vi "LSMcontroller_v60_PIzstage.vi"() -> ()   [LabVIEW 2015] (continued)
                n2600 = Unbundle By Name(w5604) -> ("Vto2P"=w5603:i32, "AOlines"=w5602:tag[])
                n2601 = local write "Vpockels"(w5598) -> ()
                n2602 = property on="Laserpower \n(%)" class="Slide (strict)"("Value"=w5600) -> ()  [unwired: 2 in, 2 out]
                n2603 = Index Array(array=w5602, index=w5603) -> (element=w5601:tag)
                n2604 = call-poly <vilib>:"DAQmx Create Virtual Channel.vi"("physical channels"=w5601) -> ("task out"=w5607:refnum<k21>, "error out"=w5606:errorcluster)  [unwired: 13 in]
                n2605 = call-poly <vilib>:"DAQmx Write.vi"("task/channels in"=w5607, "data"=w5598, "error in"=w5606) -> ("task out"=w5608:refnum<k21>, "error out"=w5609:errorcluster)  [unwired: 10 in, 1 out]
                n2606 = call <vilib>:"DAQmx Start Task.vi"("task/channels in"=w5608, "error in"=w5609) -> ("task out"=w5610:refnum<k21>, "error out"=w5611:errorcluster)  [unwired: 12 in]
                n2607 = call <vilib>:"DAQmx Stop Task.vi"("task/channels in"=w5610, "error in"=w5611) -> ("task out"=w5612:refnum<k21>, "error out"=w5613:errorcluster)  [unwired: 12 in]
                n2608 = call <vilib>:"DAQmx Clear Task.vi"("task in"=w5612, "error in"=w5613) -> ()  [unwired: 13 in, 1 out]
              }
            }
          }
          event "sealtest": Value Change {
            n2609 = event-data() -> ()  [unwired: 1 in, 6 out]
            n2610 = case shown="True" "sealtest" {
              frame False {
              }
              frame True {
                n2611 = stacked-sequence {
                  seq-local: [w5615 _ _ _ _ _] -> [_ w5648 _ w5700 _ _]
                  frame #0 {
                    n2612 = stacked-sequence {
                      tunnel: [_ w5627 _] -> w5615
                      frame #0 {
                        n2613 = call "2pparameters.vi"("command"="get") -> ("params out"=w5620:T11)  [unwired: 1 in]
                        n2614 = Unbundle By Name(w5620) -> ("autoshutter"=w5621:bool)
                        n2615 = local read "OCchecked?"() -> (w5618:bool)
                        n2616 = call "sealtestwfparams.vi"("command"="set") -> ()  [unwired: 6 in, 1 out]
                        n2617 = case shown="False" w5618 {
                          frame False {
                            n2618 = One Button Dialog(message="Is the OC gain correct?", button name ("OK")="ok") -> (true=w5622:bool)
                            n2619 = local write "OCchecked?"(w5622) -> ()
                          }
                          frame True {
                          }
                        }
                        n2620 = case shown="True" w5621 {
                          frame False {
                          }
                          frame True {
                            n2621 = call "shuttercontrol.vi"("command"="close") -> ()  [unwired: 1 in, 1 out]
                          }
                        }
                        n2622 = call "allAI-temp.vi"("command"=enum16{"get", "set", "clear", "append"}."clear") -> ()  [unwired: 3 in, 2 out]
                      }
                      frame #1 {
                        n2623 = call "sealtestwfparams.vi"("command"="get") -> ("Params out"=w5633:T24)  [unwired: 6 in]
                        n2624 = Unbundle By Name(w5633) -> ("AO parameters"=w5631:T25)
                        n2625 = Index Array(array=w5631, index=0) -> (element=w5630:T26)
                        n2626 = call "generateRampedSquareWave_fromAOparameters.vi"("AO params"=w5630) -> ("Waveform"=w5626:waveform(dbl), "wflength"=w5627:i32)
                        n2627 = Build Array(w5626) -> (w5629:waveform(dbl)[])
                        n2628 = call "waveformssealtestbuffer.vi"("AO wf in"=w5629, "command"="set") -> ()  [unwired: 1 out]
                      }
                      frame #2 {
                        n2629 = local read "Vholding (mV)"() -> (w5636:sgl)
                        n2630 = local read "Current Clamp"() -> (w5642:bool)
                        n2631 = local read "Voltage Clamp"() -> (w5641:bool)
                        n2632 = local read "OCgain"() -> (w5637:sgl)
                        n2633 = local read "CC_ICgain"() -> (w5640:dbl)
                        n2634 = local read "holdon"() -> (w5635:bool)
                        n2635 = call "patchparameters.vi"("command"="get") -> ("Params out"=w5644:T14)  [unwired: 1 in]
                        n2636 = Bundle By Name(cluster=w5644, "VC"=w5641, "CC"=w5642, "CC_icg (pA/mv)"=w5640, "VC_icg (mV/mV)"=10.0, "OCG (mV/pA)"=w5637, "OVG (mV/mV)"=0.1, "Vhold (mV)"=w5636, "holdon"=w5635) -> (w5643:T14)
                        n2637 = call "patchparameters.vi"("Params in"=w5643, "command"="set") -> ()  [unwired: 1 out]
                      }
                    }
                  }
                  frame #1 {
                    w5647 = 2
                    n2638 = call "patchparameters.vi"("command"="get") -> ("Params out"=w5655:T14)  [unwired: 1 in]
                    n2639 = Unbundle By Name(w5655) -> ("holdon"=w5654:bool, "Vhold (mV)"=w5653:sgl, "CC_icg (pA/mv)"=w5661:sgl, "CC"=w5659:bool, "VC_icg (mV/mV)"=w5660:sgl)
                    n2640 = Select(t=w5661, s=w5659, f=w5660) -> (s? t:f=w5662:sgl)
                    n2641 = To Single Precision Float(number=0.001 ("y")) -> (single precision float=w5663:sgl)
                    n2642 = Compound Arithmetic op=MULTIPLY(w5653, w5662, w5663) -> (w5657:sgl)
                    n2643 = case shown="False" w5654 {
                      tunnel: w5657 -> [_ w5675]
                      tunnel: [0.0 w5675] -> w5650
                      frame False {
                      }
                      frame True {
                      }
                    }
                    n2644 = Greater Than 0?(x=w5647) -> (x > 0?=w5649:bool)
                    n2645 = case shown="True" w5649 {
                      tunnel: w5648 -> [_ w5664]
                      tunnel: w5647 -> [_ w5667]
                      frame False {
                      }
                      frame True {
                        n2646 = Initialize Array(sgl 0.0 ("element"), w5667, w5664) -> (w5665:sgl[][])
                        n2647 = call "allAI-temp.vi"("array in"=w5665, "command"=enum16{"get", "set", "clear", "append"}."set") -> ()  [unwired: 2 in, 2 out]
                      }
                    }
                    n2648 = flat-sequence {
                      tunnel: w5648 -> [w5671]
                      tunnel: w5648 -> [w5670]
                      tunnel: [w5670] -> w5652
                      tunnel: [w5669] -> w5651
                      tunnel: w5650 -> [w5669]
                      tunnel: w5652 -> [w5673]
                      tunnel: w5651 -> [w5672]
                      frame #0 {
                        n2649 = call "prepAI_sealtest.vi"("samples per channel"=w5671) -> ()  [unwired: 2 in]
                      }
                      frame #1 {
                        n2650 = call "prepAO_sealtest.vi"("Vhold"=w5672, "samples per channel"=w5673) -> ()  [unwired: 1 in]
                      }
                    }
                  }
                  frame #2 {
                    n2651 = stacked-sequence {
                      frame #0 {
                        n2652 = call "tempconfigAO.vi"("command"="get") -> ("Temp Config out"=w5679:T27)  [unwired: 1 in]
                        n2653 = Unbundle By Name(w5679) -> ("AO"=w5680:refnum<k21>[], "E_AO"=w5681:errorcluster[])
                        n2654 = for {
                          tunnel: w5680 -> [w5689] mode=indexing
                          tunnel: w5681 -> [w5688] mode=indexing
                          tunnel: [w5687] -> w5683 mode=indexing
                          tunnel: [w5686] -> w5684 mode=indexing
                          n2655 = call <vilib>:"DAQmx Start Task.vi"("task/channels in"=w5689, "error in"=w5688) -> ("task out"=w5687:refnum<k21>, "error out"=w5686:errorcluster)  [unwired: 12 in]
                        }
                        n2656 = call "tempconfigAO.vi"("command"="get") -> ("Temp Config out"=w5682:T27)  [unwired: 1 in]
                        n2657 = Bundle By Name(cluster=w5682, "AO"=w5683, "E_AO"=w5684) -> (w5685:T27)
                        n2658 = call "tempconfigAO.vi"("Temp Config in"=w5685, "command"="set") -> ()  [unwired: 1 out]
                      }
                      frame #1 {
                        n2659 = call "tempconfigAI.vi"("command"="get") -> ("Temp Config out"=w5691:T28)  [unwired: 1 in]
                        n2660 = Unbundle By Name(w5691) -> ("AI"=w5696:refnum<k21>, "E_AI"=w5697:errorcluster)
                        n2661 = call <vilib>:"DAQmx Start Task.vi"("task/channels in"=w5696, "error in"=w5697) -> ("task out"=w5698:refnum<k21>, "error out"=w5699:errorcluster)  [unwired: 12 in]
                        n2662 = call "tempconfigAI.vi"("command"="get") -> ("Temp Config out"=w5693:T28)  [unwired: 1 in]
                        n2663 = Bundle By Name(cluster=w5693, "AI"=w5698, "E_AI"=w5699) -> (w5695:T28)
                        n2664 = call "tempconfigAI.vi"("Temp Config in"=w5695, "command"="set") -> ()  [unwired: 1 out]
                      }
                    }
                  }
                  frame #3 {
                    n2665 = while {
                      tunnel: w5700 -> [w5701]
                      stop <- w5702 stop-if-true
                      n2666 = local read "sealtest"() -> (w5705:bool)
                      n2667 = Not(x=w5705) -> (.not. x?=w5704:bool)
                      n2668 = case shown="False" w5704 {
                        tunnel: w5701 -> [w5706 _]
                        frame False {
                          n2669 = stacked-sequence {
                            seq-local: [_ _ _ w5745 _ _] -> [_ _ _ _ w5801 _]
                            seq-local: [w5707 _ _ _ _ _] -> [_ w5716 _ w5738 w5790 w5821]
                            tunnel: w5706 -> [_ _ w5724 _ w5789 _]
                            frame #0 {
                              n2670 = call "patchparameters.vi"("command"="get") -> ("Params out"=w5714:T14)  [unwired: 1 in]
                              n2671 = local read "Vholding (mV)"() -> (w5711:sgl)
                              n2672 = Unbundle By Name(w5714) -> ("Vhold (mV)"=w5710:sgl, "holdon"=w5713:bool)
                              n2673 = local read "holdon"() -> (w5712:bool)
                              n2674 = Not Equal?(x=w5711, y=w5710) -> (x != y?=w5709:bool)
                              n2675 = Not Equal?(x=w5713, y=w5712) -> (x != y?=w5708:bool)
                              n2676 = Or(x=w5709, y=w5708) -> (x .or. y?=w5707:bool)
                            }
                            frame #1 {
                              n2677 = case shown="True" w5716 {
                                frame False {
                                }
                                frame True {
                                n2678 = local read "Vholding (mV)"() -> (w5719:sgl)
                                n2679 = local read "holdon"() -> (w5717:bool)
                                n2680 = call "patchparameters.vi"("command"="get") -> ("Params out"=w5720:T14)  [unwired: 1 in]
                                n2681 = Bundle By Name(cluster=w5720, "Vhold (mV)"=w5719, "holdon"=w5717) -> (w5718:T14)
                                n2682 = call "patchparameters.vi"("Params in"=w5718, "command"="set") -> ()  [unwired: 1 out]
                                }
                              }
                            }
                            frame #2 {
                              n2683 = call "tempconfigAI.vi"("command"="get") -> ("Temp Config out"=w5734:T28)  [unwired: 1 in]
                              n2684 = Unbundle By Name(w5734) -> ("AI"=w5733:refnum<k21>, "E_AI"=w5732:errorcluster)
                              n2685 = call-poly <vilib>:"DAQmx Read.vi"("task/channels in"=w5733, "number of samples per channel"=w5724, "timeout"=10.0, "error in"=w5732) -> ("task out"=w5728:refnum<k21>, "data"=w5725:i16[][], "error out"=w5737:errorcluster)  [unwired: 9 in]
                              n2686 = call "tempconfigAI.vi"("command"="get") -> ("Temp Config out"=w5729:T28)  [unwired: 1 in]
                              n2687 = Bundle By Name(cluster=w5729, "AI"=w5728, "E_AI"=w5737) -> (w5736:T28)
                              n2688 = To Single Precision Float(number=w5725) -> (single precision float=w5727:sgl[][])
                              n2689 = call "tempconfigAI.vi"("Temp Config in"=w5736, "command"="set") -> ()  [unwired: 1 out]
                              n2690 = call "allAI-temp.vi"("array in"=w5727, "command"=enum16{"get", "set", "clear", "append"}."set") -> ()  [unwired: 2 in, 2 out]
                            }
                            frame #3 {
                              n2691 = case shown="True" w5738 {
                                frame False {
                                }
                                frame True {
                                n2692 = call "tempconfigAO.vi"("command"="get") -> ("Temp Config out"=w5778:T27)  [unwired: 1 in]
                                n2693 = Unbundle By Name(w5778) -> ("AO"=w5777:refnum<k21>[], "E_AO"=w5776:errorcluster[])
                                n2694 = call "tempconfigAI.vi"("command"="get") -> ("Temp Config out"=w5765:T28)  [unwired: 1 in]
                                n2695 = Unbundle By Name(w5765) -> ("AI"=w5766:refnum<k21>, "E_AI"=w5767:errorcluster)
                                n2696 = for {
                                tunnel: w5777 -> [w5782] mode=indexing
                                tunnel: w5776 -> [w5781] mode=indexing
                                tunnel: [w5780] -> w5772 mode=indexing
                                n2697 = call <vilib>:"DAQmx Stop Task.vi"("task/channels in"=w5782, "error in"=w5781) -> ("task out"=w5783:refnum<k21>, "error out"=w5784:errorcluster)  [unwired: 12 in]
                                n2698 = call <vilib>:"DAQmx Clear Task.vi"("task in"=w5783, "error in"=w5784) -> ("error out"=w5780:errorcluster)  [unwired: 13 in]
                                }
                                n2699 = call <vilib>:"DAQmx Stop Task.vi"("task/channels in"=w5766, "error in"=w5767) -> ("task out"=w5763:refnum<k21>, "error out"=w5762:errorcluster)  [unwired: 12 in]
                                n2700 = call <vilib>:"DAQmx Clear Task.vi"("task in"=w5763, "error in"=w5762) -> ("error out"=w5761:errorcluster)  [unwired: 13 in]
                                n2701 = call "tempconfigAO.vi"("command"="get") -> ("Temp Config out"=w5773:T27)  [unwired: 1 in]
                                n2702 = Bundle By Name(cluster=w5773, "E_AO"=w5772) -> (w5771:T27)
                                n2703 = call "tempconfigAI.vi"("command"="get") -> ("Temp Config out"=w5769:T28)  [unwired: 1 in]
                                n2704 = Bundle By Name(cluster=w5769, "E_AI"=w5761) -> (w5760:T28)
                                n2705 = call "tempconfigAO.vi"("Temp Config in"=w5771, "command"="set") -> ()  [unwired: 1 out]
                                n2706 = call "tempconfigAI.vi"("Temp Config in"=w5760, "command"="set") -> ()  [unwired: 1 out]
                                }
                              }
                              n2707 = call "allAI-temp.vi"("command"=enum16{"get", "set", "clear", "append"}."get") -> ("array out"=w5742:sgl[][])  [unwired: 3 in, 1 out]
                              n2708 = call "tempconfigAI.vi"("command"="get") -> ("Temp Config out"=w5755:T28)  [unwired: 1 in]
                              n2709 = call "tempconfigAI.vi"("command"="get") -> ("Temp Config out"=w5757:T28)  [unwired: 1 in]
                              n2710 = Unbundle By Name(w5755) -> ("header"=w5753:dbl[])
                              n2711 = Unbundle By Name(w5757) -> ("header"=w5759:dbl[])
                              n2712 = Index Array(array=w5742, index (row) #1=1 ("index (row)"), index (row) #2=0 ("index (row)")) -> (element #1=w5740:sgl[], element #2=w5739:sgl[])  [unwired: 2 in]
                              n2713 = local read "OCgain"() -> (w5747:sgl)
                              n2714 = call "Unscaledtoscaled.vi"("Unscaled Data"=w5740, "Header Information"=w5753) -> ("Array"=w5752:sgl[])  [unwired: 1 in]
                              n2715 = call "Unscaledtoscaled.vi"("Unscaled Data"=w5739, "Header Information"=w5759) -> ("Array"=w5756:sgl[])  [unwired: 1 in]
                              n2716 = Multiply(x=w5752, y=0.1) -> (x*y=w5749:dbl[])
                              n2717 = Divide(x=w5756, y=w5747) -> (x/y=w5748:sgl[])
                              n2718 = Build Array(w5749, w5748) -> (w5751:dbl[][])
                              n2719 = Multiply(x=w5751, y=1000.0) -> (x*y=w5745:dbl[][])
                              "Patch readout" <- w5745
                            }
                            frame #4 {
                              n2720 = case shown="True" w5790 {
                                tunnel: w5789 -> [_ w5802]
                                frame False {
                                }
                                frame True {
                                n2721 = call "patchparameters.vi"("command"="get") -> ("Params out"=w5806:T14)  [unwired: 1 in]
                                n2722 = Unbundle By Name(w5806) -> ("holdon"=w5805:bool, "Vhold (mV)"=w5804:sgl, "CC_icg (pA/mv)"=w5812:sgl, "CC"=w5810:bool, "VC_icg (mV/mV)"=w5811:sgl)
                                n2723 = Select(t=w5812, s=w5810, f=w5811) -> (s? t:f=w5813:sgl)
                                n2724 = To Single Precision Float(number=0.001 ("y")) -> (single precision float=w5814:sgl)
                                n2725 = Compound Arithmetic op=MULTIPLY(w5804, w5813, w5814) -> (w5808:sgl)
                                n2726 = case shown="True" w5805 {
                                tunnel: w5808 -> [_ w5819]
                                tunnel: [0.0 w5819] -> w5803
                                frame False {
                                }
                                frame True {
                                }
                                }
                                n2727 = flat-sequence {
                                tunnel: w5802 -> [w5815]
                                tunnel: w5803 -> [w5817]
                                tunnel: w5802 -> [w5816]
                                frame #0 {
                                n2728 = call "prepAI_sealtest.vi"("samples per channel"=w5815) -> ()  [unwired: 2 in]
                                }
                                frame #1 {
                                n2729 = call "prepAO_sealtest.vi"("Vhold"=w5817, "samples per channel"=w5816) -> ()  [unwired: 1 in]
                                }
                                }
                                }
                              }
                              n2730 = call "sealtestwfparams.vi"("command"="get") -> ("Params out"=w5795:T24)  [unwired: 6 in]
                              n2731 = Unbundle By Name(w5795) -> ("AO parameters"=w5796:T25)
                              n2732 = Index Array(array=w5796, index=0) -> (element=w5798:T26)
                              n2733 = Unbundle By Name(w5798) -> ("Cycles"=w5793:dbl, "Start amplitude (V)"=w5792:dbl, "Sampling frequency (Hz)"=w5791:dbl)
                              n2734 = local read "fitpoints"() -> (w5799:dbl)
                              n2735 = script code="V=data(1,:);\nI=data(2,:);\ntres=mean(V);\nspc=(nsamp./ncyc);\nV=V(spc+1:end-spc);\nI=I(spc+1:end-spc);\ndV=mean(V(V>tres))-mean(V(V<tres))\nIcyc=reshape(I,[spc ncyc-2]);\nIcyc=Icyc';\nIcyc=mean(Icyc,1);\ndIss=mean(Icyc(floor(spc*0.15):floor(spc/2)-2))-mean(Icyc(spc*0.65:spc-2))\nRm=dV*1e3/dIss;\n[maxi,ind]=max(Icyc);\nIfit=Icyc(ind+1:ind+1+points-1)-0.5*(mean(Icyc(floor(spc*0.15):floor(spc/2)-2))+mean(Icyc(spc*0.65:spc-2)))\nt=(3:points-1+3)./srate*1000;\nt=t';\nIfit=Ifit';\nc=fit(t,Ifit, 'exp1');\ncoeffs=coeffvalues(c);\nIa=coeffs(1);\nRa=dV*1e3./Ia/2;\ntau=-1./coeffs(2);\ncap=tau/Ra*1000;"("data"=w5801, "nsamp"=w5789, "ncyc"=w5793, "maxV"=w5792, "points"=w5799, "srate"=w5791) -> ("cap"=w5788:dbl, "Ra"=w5787:dbl, "Icyc"=w5786:dbl[], "Rm"=w5785:dbl)  [unwired: 1 in, 1 out]
                              n2736 = local read "set as Rp?"() -> (w5800:bool)
                              n2737 = local write "Cmembrane"(w5788) -> ()
                              n2738 = local write "Rmembrane (MOhm)"(w5785) -> ()
                              n2739 = local write "Racces (MOhm)"(w5787) -> ()
                              n2740 = case shown="True" w5800 {
                                tunnel: w5785 -> [_ w5820]
                                frame False {
                                }
                                frame True {
                                n2741 = local write "Rpipette (MOhm)"(w5820) -> ()
                                }
                              }
                              n2742 = local write "Ifit"(w5786) -> ()
                            }
                            frame #5 {
                              n2743 = local read "set as Rp?"() -> (w5822:bool)
                              n2744 = case shown="True" w5821 {
                                frame False {
                                }
                                frame True {
                                n2745 = stacked-sequence {
                                frame #0 {
                                n2746 = call "tempconfigAO.vi"("command"="get") -> ("Temp Config out"=w5829:T27)  [unwired: 1 in]
                                n2747 = Unbundle By Name(w5829) -> ("AO"=w5828:refnum<k21>[], "E_AO"=w5827:errorcluster[])
                                n2748 = for {
                                tunnel: w5828 -> [w5836] mode=indexing
                                tunnel: w5827 -> [w5835] mode=indexing
                                tunnel: [w5834] -> w5825 mode=indexing
                                tunnel: [w5833] -> w5824 mode=indexing
                                n2749 = call <vilib>:"DAQmx Start Task.vi"("task/channels in"=w5836, "error in"=w5835) -> ("task out"=w5834:refnum<k21>, "error out"=w5833:errorcluster)  [unwired: 12 in]
                                }
                                n2750 = call "tempconfigAO.vi"("command"="get") -> ("Temp Config out"=w5826:T27)  [unwired: 1 in]
                                n2751 = Bundle By Name(cluster=w5826, "AO"=w5825, "E_AO"=w5824) -> (w5823:T27)
                                n2752 = call "tempconfigAO.vi"("Temp Config in"=w5823, "command"="set") -> ()  [unwired: 1 out]
                                }
                                frame #1 {
                                n2753 = call "tempconfigAI.vi"("command"="get") -> ("Temp Config out"=w5838:T28)  [unwired: 1 in]
                                n2754 = Unbundle By Name(w5838) -> ("AI"=w5843:refnum<k21>, "E_AI"=w5844:errorcluster)
                                n2755 = call <vilib>:"DAQmx Start Task.vi"("task/channels in"=w5843, "error in"=w5844) -> ("task out"=w5845:refnum<k21>, "error out"=w5846:errorcluster)  [unwired: 12 in]
                                n2756 = call "tempconfigAI.vi"("command"="get") -> ("Temp Config out"=w5840:T28)  [unwired: 1 in]
                                n2757 = Bundle By Name(cluster=w5840, "AI"=w5845, "E_AI"=w5846) -> (w5842:T28)
                                n2758 = call "tempconfigAI.vi"("Temp Config in"=w5842, "command"="set") -> ()  [unwired: 1 out]
                                }
                                }
                                }
                              }
                              n2759 = case shown="True" w5822 {
                                frame False {
                                }
                                frame True {
                                n2760 = local write "set as Rp?"(FALSE ("set as Rp?")) -> ()
                                }
                              }
                            }
                          }
                        }
                        frame True {
                        }
                      }
                      n2761 = local read "sealtest"() -> (w5703:bool)
                      n2762 = Not(x=w5703) -> (.not. x?=w5702:bool)
                    }
                  }
                  frame #4 {
                    n2763 = call "tempconfigAO.vi"("command"="get") -> ("Temp Config out"=w5873:T27)  [unwired: 1 in]
                    n2764 = Unbundle By Name(w5873) -> ("AO"=w5872:refnum<k21>[], "E_AO"=w5871:errorcluster[])
                    n2765 = call "configuration.vi"("command"="get") -> ("config out"=w5854:T12)  [unwired: 2 in, 1 out]
                    n2766 = call "tempconfigAI.vi"("command"="get") -> ("Temp Config out"=w5860:T28)  [unwired: 1 in]
                    n2767 = Unbundle By Name(w5854) -> ("Device 1 sampleclock out"=w5851:tag, "Device 1 Starttrigger out"=w5850:tag)
                    n2768 = Unbundle By Name(w5860) -> ("AI"=w5861:refnum<k21>, "E_AI"=w5862:errorcluster)
                    n2769 = for {
                      tunnel: w5872 -> [w5877] mode=indexing
                      tunnel: w5871 -> [w5876] mode=indexing
                      tunnel: [w5875] -> w5867 mode=indexing
                      n2770 = call <vilib>:"DAQmx Stop Task.vi"("task/channels in"=w5877, "error in"=w5876) -> ("task out"=w5878:refnum<k21>, "error out"=w5879:errorcluster)  [unwired: 12 in]
                      n2771 = call <vilib>:"DAQmx Clear Task.vi"("task in"=w5878, "error in"=w5879) -> ("error out"=w5875:errorcluster)  [unwired: 13 in]
                    }
                    n2772 = call <vilib>:"DAQmx Stop Task.vi"("task/channels in"=w5861, "error in"=w5862) -> ("task out"=w5858:refnum<k21>, "error out"=w5857:errorcluster)  [unwired: 12 in]
                    n2773 = call <vilib>:"DAQmx Disconnect Terminals.vi"("source terminal"=tag "/Dev1/ai/SampleClock", "destination terminal"=w5851) -> ("error out"=w5848:errorcluster)  [unwired: 13 in]
                    n2774 = call <vilib>:"DAQmx Clear Task.vi"("task in"=w5858, "error in"=w5857) -> ("error out"=w5856:errorcluster)  [unwired: 13 in]
                    n2775 = call "tempconfigAO.vi"("command"="get") -> ("Temp Config out"=w5868:T27)  [unwired: 1 in]
                    n2776 = Bundle By Name(cluster=w5868, "E_AO"=w5867) -> (w5866:T27)
                    n2777 = call "tempconfigAI.vi"("command"="get") -> ("Temp Config out"=w5864:T28)  [unwired: 1 in]
                    n2778 = Bundle By Name(cluster=w5864, "E_AI"=w5856) -> (w5855:T28)
                    n2779 = call "tempconfigAO.vi"("Temp Config in"=w5866, "command"="set") -> ()  [unwired: 1 out]
                    n2780 = call <vilib>:"DAQmx Disconnect Terminals.vi"("source terminal"=tag "/Dev1/ai/StartTrigger", "destination terminal"=w5850, "error in"=w5848) -> ()  [unwired: 12 in, 1 out]
                    n2781 = call "tempconfigAI.vi"("Temp Config in"=w5855, "command"="set") -> ()  [unwired: 1 out]
                  }
                  frame #5 {
                    w5882 = T22 4 items=["no dialog", "OK message", "continue or stop message", "OK message + warnings", "continue/stop + warnings"] ("type of dialog (OK msg:1)")
                    n2782 = call "displayerrors.vi"() -> ("error IO"=w5881:errorcluster)
                    n2783 = call "zeropatch.vi"() -> ()  [unwired: 12 in]
                    n2784 = call <vilib>:"Simple Error Handler.vi"("type of dialog (OK msg:1)"=w5882, "error in (no error)"=w5881) -> ("error out"=w5880:errorcluster)  [unwired: 3 in, 4 out]
                    n2785 = call <vilib>:"Clear Errors.vi"("error in (no error)"=w5880) -> ()  [unwired: 5 in, 2 out]
                  }
                }
              }
            }
          }
          event "readpatch": Value Change {
            n2786 = event-data() -> ()  [unwired: 1 in, 6 out]
            n2787 = local read "readpatch"() -> (w5883:bool)
            n2788 = case shown="True" w5883 {
              frame False {
              }
              frame True {
                n2789 = stacked-sequence {
                  seq-local: [w5884 _ _ _ _ _] -> [_ w5917 _ w5969 _ _]
                  frame #0 {
                    n2790 = stacked-sequence {
                      tunnel: [_ w5896 _] -> w5884
                      frame #0 {
                        n2791 = call "2pparameters.vi"("command"="get") -> ("params out"=w5889:T11)  [unwired: 1 in]
                        n2792 = Unbundle By Name(w5889) -> ("autoshutter"=w5890:bool)
                        n2793 = local read "OCchecked?"() -> (w5887:bool)
                        n2794 = call "sealtestwfparams.vi"("command"="set") -> ()  [unwired: 6 in, 1 out]
                        n2795 = case shown="False" w5887 {
                          frame False {
                            n2796 = One Button Dialog(message="Is the OC gain correct?", button name ("OK")="ok") -> (true=w5891:bool)
                            n2797 = local write "OCchecked?"(w5891) -> ()
                          }
                          frame True {
                          }
                        }
                        n2798 = case shown="True" w5890 {
                          frame False {
                          }
                          frame True {
                            n2799 = call "shuttercontrol.vi"("command"="close") -> ()  [unwired: 1 in, 1 out]
                          }
                        }
                        n2800 = call "allAI-temp.vi"("command"=enum16{"get", "set", "clear", "append"}."clear") -> ()  [unwired: 3 in, 2 out]
                      }
                      frame #1 {
                        n2801 = call "sealtestwfparams.vi"("command"="get") -> ("Params out"=w5902:T24)  [unwired: 6 in]
                        n2802 = Unbundle By Name(w5902) -> ("AO parameters"=w5900:T25)
                        n2803 = Index Array(array=w5900, index=1) -> (element=w5899:T26)
                        n2804 = call "generateRampedSquareWave_fromAOparameters.vi"("AO params"=w5899) -> ("Waveform"=w5895:waveform(dbl), "wflength"=w5896:i32)
                        n2805 = Build Array(w5895) -> (w5898:waveform(dbl)[])
                        n2806 = call "waveformssealtestbuffer.vi"("AO wf in"=w5898, "command"="set") -> ()  [unwired: 1 out]
                      }
                      frame #2 {
                        n2807 = local read "Vholding (mV)"() -> (w5905:sgl)
                        n2808 = local read "Current Clamp"() -> (w5911:bool)
                        n2809 = local read "Voltage Clamp"() -> (w5910:bool)
                        n2810 = local read "OCgain"() -> (w5906:sgl)
                        n2811 = local read "CC_ICgain"() -> (w5909:dbl)
                        n2812 = local read "holdon"() -> (w5904:bool)
                        n2813 = call "patchparameters.vi"("command"="get") -> ("Params out"=w5913:T14)  [unwired: 1 in]
                        n2814 = Bundle By Name(cluster=w5913, "VC"=w5910, "CC"=w5911, "CC_icg (pA/mv)"=w5909, "VC_icg (mV/mV)"=10.0, "OCG (mV/pA)"=w5906, "OVG (mV/mV)"=0.1, "Vhold (mV)"=w5905, "holdon"=w5904) -> (w5912:T14)
                        n2815 = call "patchparameters.vi"("Params in"=w5912, "command"="set") -> ()  [unwired: 1 out]
                      }
                    }
                  }
                  frame #1 {
                    w5916 = 2
                    n2816 = call "patchparameters.vi"("command"="get") -> ("Params out"=w5924:T14)  [unwired: 1 in]
                    n2817 = Unbundle By Name(w5924) -> ("holdon"=w5923:bool, "Vhold (mV)"=w5922:sgl, "CC_icg (pA/mv)"=w5930:sgl, "CC"=w5928:bool, "VC_icg (mV/mV)"=w5929:sgl)
                    n2818 = Select(t=w5930, s=w5928, f=w5929) -> (s? t:f=w5931:sgl)
                    n2819 = To Single Precision Float(number=0.001 ("y")) -> (single precision float=w5932:sgl)
                    n2820 = Compound Arithmetic op=MULTIPLY(w5922, w5931, w5932) -> (w5926:sgl)
                    n2821 = case shown="False" w5923 {
                      tunnel: w5926 -> [_ w5944]
                      tunnel: [0.0 w5944] -> w5919
                      frame False {
                      }
                      frame True {
                      }
                    }
                    n2822 = Greater Than 0?(x=w5916) -> (x > 0?=w5918:bool)
                    n2823 = case shown="True" w5918 {
                      tunnel: w5917 -> [_ w5933]
                      tunnel: w5916 -> [_ w5936]
                      frame False {
                      }
                      frame True {
                        n2824 = Initialize Array(sgl 0.0 ("element"), w5936, w5933) -> (w5934:sgl[][])
                        n2825 = call "allAI-temp.vi"("array in"=w5934, "command"=enum16{"get", "set", "clear", "append"}."set") -> ()  [unwired: 2 in, 2 out]
                      }
                    }
                    n2826 = flat-sequence {
                      tunnel: w5917 -> [w5940]
                      tunnel: w5917 -> [w5939]
                      tunnel: [w5939] -> w5921
                      tunnel: [w5938] -> w5920
                      tunnel: w5919 -> [w5938]
                      tunnel: w5921 -> [w5942]
                      tunnel: w5920 -> [w5941]
                      frame #0 {
                        n2827 = call "prepAI_sealtest.vi"("samples per channel"=w5940) -> ()  [unwired: 2 in]
                      }
                      frame #1 {
                        n2828 = call "prepAO_sealtest.vi"("Vhold"=w5941, "samples per channel"=w5942) -> ()  [unwired: 1 in]
                      }
                    }
                  }
                  frame #2 {
                    n2829 = stacked-sequence {
                      frame #0 {
                        n2830 = call "tempconfigAO.vi"("command"="get") -> ("Temp Config out"=w5948:T27)  [unwired: 1 in]
                        n2831 = Unbundle By Name(w5948) -> ("AO"=w5949:refnum<k21>[], "E_AO"=w5950:errorcluster[])
                        n2832 = for {
                          tunnel: w5949 -> [w5958] mode=indexing
                          tunnel: w5950 -> [w5957] mode=indexing
                          tunnel: [w5956] -> w5952 mode=indexing
                          tunnel: [w5955] -> w5953 mode=indexing
                          n2833 = call <vilib>:"DAQmx Start Task.vi"("task/channels in"=w5958, "error in"=w5957) -> ("task out"=w5956:refnum<k21>, "error out"=w5955:errorcluster)  [unwired: 12 in]
                        }
                        n2834 = call "tempconfigAO.vi"("command"="get") -> ("Temp Config out"=w5951:T27)  [unwired: 1 in]
                        n2835 = Bundle By Name(cluster=w5951, "AO"=w5952, "E_AO"=w5953) -> (w5954:T27)
                        n2836 = call "tempconfigAO.vi"("Temp Config in"=w5954, "command"="set") -> ()  [unwired: 1 out]
                      }
                      frame #1 {
                        n2837 = call "tempconfigAI.vi"("command"="get") -> ("Temp Config out"=w5960:T28)  [unwired: 1 in]
                        n2838 = Unbundle By Name(w5960) -> ("AI"=w5965:refnum<k21>, "E_AI"=w5966:errorcluster)
                        n2839 = call <vilib>:"DAQmx Start Task.vi"("task/channels in"=w5965, "error in"=w5966) -> ("task out"=w5967:refnum<k21>, "error out"=w5968:errorcluster)  [unwired: 12 in]
                        n2840 = call "tempconfigAI.vi"("command"="get") -> ("Temp Config out"=w5962:T28)  [unwired: 1 in]
                        n2841 = Bundle By Name(cluster=w5962, "AI"=w5967, "E_AI"=w5968) -> (w5964:T28)
                        n2842 = call "tempconfigAI.vi"("Temp Config in"=w5964, "command"="set") -> ()  [unwired: 1 out]
                      }
                    }
                  }
                  frame #3 {
                    n2843 = while {
                      tunnel: w5969 -> [w5970]
                      stop <- w5971 stop-if-true
                      n2844 = local read "readpatch"() -> (w5974:bool)
                      n2845 = Not(x=w5974) -> (.not. x?=w5973:bool)
                      n2846 = case shown="True" w5973 {
                        tunnel: w5970 -> [w5975 _]
                        frame False {
                          n2847 = stacked-sequence {
                            seq-local: [w5976 _ _ _ _ _] -> [_ w5985 _ w6008 w6055 w6074]
                            tunnel: w5975 -> [_ _ w5993 _ w6054 _]
                            frame #0 {
                              n2848 = call "patchparameters.vi"("command"="get") -> ("Params out"=w5983:T14)  [unwired: 1 in]
                              n2849 = local read "Vholding (mV)"() -> (w5980:sgl)
                              n2850 = Unbundle By Name(w5983) -> ("Vhold (mV)"=w5979:sgl, "holdon"=w5982:bool)
                              n2851 = local read "holdon"() -> (w5981:bool)
                              n2852 = Not Equal?(x=w5980, y=w5979) -> (x != y?=w5978:bool)
                              n2853 = Not Equal?(x=w5982, y=w5981) -> (x != y?=w5977:bool)
                              n2854 = Or(x=w5978, y=w5977) -> (x .or. y?=w5976:bool)
                            }
                            frame #1 {
                              n2855 = case shown="False" w5985 {
                                frame False {
                                }
                                frame True {
                                n2856 = local read "Vholding (mV)"() -> (w5988:sgl)
                                n2857 = local read "holdon"() -> (w5986:bool)
                                n2858 = call "patchparameters.vi"("command"="get") -> ("Params out"=w5989:T14)  [unwired: 1 in]
                                n2859 = Bundle By Name(cluster=w5989, "Vhold (mV)"=w5988, "holdon"=w5986) -> (w5987:T14)
                                n2860 = call "patchparameters.vi"("Params in"=w5987, "command"="set") -> ()  [unwired: 1 out]
                                }
                              }
                            }
                            frame #2 {
                              n2861 = call "tempconfigAI.vi"("command"="get") -> ("Temp Config out"=w6003:T28)  [unwired: 1 in]
                              n2862 = Unbundle By Name(w6003) -> ("AI"=w6002:refnum<k21>, "E_AI"=w6001:errorcluster)
                              n2863 = call-poly <vilib>:"DAQmx Read.vi"("task/channels in"=w6002, "number of samples per channel"=w5993, "timeout"=10.0, "error in"=w6001) -> ("task out"=w5997:refnum<k21>, "data"=w5994:i16[][], "error out"=w6006:errorcluster)  [unwired: 9 in]
                              n2864 = call "tempconfigAI.vi"("command"="get") -> ("Temp Config out"=w5998:T28)  [unwired: 1 in]
                              n2865 = Bundle By Name(cluster=w5998, "AI"=w5997, "E_AI"=w6006) -> (w6005:T28)
                              n2866 = To Single Precision Float(number=w5994) -> (single precision float=w5996:sgl[][])
                              n2867 = call "tempconfigAI.vi"("Temp Config in"=w6005, "command"="set") -> ()  [unwired: 1 out]
                              n2868 = call "allAI-temp.vi"("array in"=w5996, "command"=enum16{"get", "set", "clear", "append"}."set") -> ()  [unwired: 2 in, 2 out]
                            }
                            frame #3 {
                              n2869 = case shown="True" w6008 {
                                frame False {
                                }
                                frame True {
                                n2870 = call "tempconfigAO.vi"("command"="get") -> ("Temp Config out"=w6047:T27)  [unwired: 1 in]
                                n2871 = Unbundle By Name(w6047) -> ("AO"=w6046:refnum<k21>[], "E_AO"=w6045:errorcluster[])
                                n2872 = call "tempconfigAI.vi"("command"="get") -> ("Temp Config out"=w6034:T28)  [unwired: 1 in]
                                n2873 = Unbundle By Name(w6034) -> ("AI"=w6035:refnum<k21>, "E_AI"=w6036:errorcluster)
                                n2874 = for {
                                tunnel: w6046 -> [w6051] mode=indexing
                                tunnel: w6045 -> [w6050] mode=indexing
                                tunnel: [w6049] -> w6041 mode=indexing
                                n2875 = call <vilib>:"DAQmx Stop Task.vi"("task/channels in"=w6051, "error in"=w6050) -> ("task out"=w6052:refnum<k21>, "error out"=w6053:errorcluster)  [unwired: 12 in]
                                n2876 = call <vilib>:"DAQmx Clear Task.vi"("task in"=w6052, "error in"=w6053) -> ("error out"=w6049:errorcluster)  [unwired: 13 in]
                                }
                                n2877 = call <vilib>:"DAQmx Stop Task.vi"("task/channels in"=w6035, "error in"=w6036) -> ("task out"=w6032:refnum<k21>, "error out"=w6031:errorcluster)  [unwired: 12 in]
                                n2878 = call <vilib>:"DAQmx Clear Task.vi"("task in"=w6032, "error in"=w6031) -> ("error out"=w6030:errorcluster)  [unwired: 13 in]
                                n2879 = call "tempconfigAO.vi"("command"="get") -> ("Temp Config out"=w6042:T27)  [unwired: 1 in]
                                n2880 = Bundle By Name(cluster=w6042, "E_AO"=w6041) -> (w6040:T27)
                                n2881 = call "tempconfigAI.vi"("command"="get") -> ("Temp Config out"=w6038:T28)  [unwired: 1 in]
                                n2882 = Bundle By Name(cluster=w6038, "E_AI"=w6030) -> (w6029:T28)
                                n2883 = call "tempconfigAO.vi"("Temp Config in"=w6040, "command"="set") -> ()  [unwired: 1 out]
                                n2884 = call "tempconfigAI.vi"("Temp Config in"=w6029, "command"="set") -> ()  [unwired: 1 out]
                                }
                              }
                              n2885 = call "allAI-temp.vi"("command"=enum16{"get", "set", "clear", "append"}."get") -> ("array out"=w6012:sgl[][])  [unwired: 3 in, 1 out]
                              n2886 = call "tempconfigAI.vi"("command"="get") -> ("Temp Config out"=w6024:T28)  [unwired: 1 in]
                              n2887 = call "tempconfigAI.vi"("command"="get") -> ("Temp Config out"=w6026:T28)  [unwired: 1 in]
                              n2888 = Unbundle By Name(w6024) -> ("header"=w6022:dbl[])
                              n2889 = Unbundle By Name(w6026) -> ("header"=w6028:dbl[])
                              n2890 = Index Array(array=w6012, index (row) #1=1 ("index (row)"), index (row) #2=0 ("index (row)")) -> (element #1=w6010:sgl[], element #2=w6009:sgl[])  [unwired: 2 in]
                              n2891 = local read "OCgain"() -> (w6016:sgl)
                              n2892 = call "Unscaledtoscaled.vi"("Unscaled Data"=w6010, "Header Information"=w6022) -> ("Array"=w6021:sgl[])  [unwired: 1 in]
                              n2893 = call "Unscaledtoscaled.vi"("Unscaled Data"=w6009, "Header Information"=w6028) -> ("Array"=w6025:sgl[])  [unwired: 1 in]
                              n2894 = Multiply(x=w6021, y=0.1) -> (x*y=w6018:dbl[])
                              n2895 = Divide(x=w6025, y=w6016) -> (x/y=w6017:sgl[])
                              n2896 = Build Array(w6018, w6017) -> (w6020:dbl[][])
                              n2897 = Multiply(x=w6020, y=1000.0) -> (x*y=w6007:dbl[][])
                              n2898 = local write "Patch readout"(w6007) -> ()
                            }
                            frame #4 {
                              n2899 = case shown="True" w6055 {
                                tunnel: w6054 -> [_ w6056]
                                frame False {
                                }
                                frame True {
                                n2900 = call "patchparameters.vi"("command"="get") -> ("Params out"=w6060:T14)  [unwired: 1 in]
                                n2901 = Unbundle By Name(w6060) -> ("holdon"=w6059:bool, "Vhold (mV)"=w6058:sgl, "CC_icg (pA/mv)"=w6066:sgl, "CC"=w6064:bool, "VC_icg (mV/mV)"=w6065:sgl)
                                n2902 = Select(t=w6066, s=w6064, f=w6065) -> (s? t:f=w6067:sgl)
                                n2903 = To Single Precision Float(number=0.001 ("y")) -> (single precision float=w6068:sgl)
                                n2904 = Compound Arithmetic op=MULTIPLY(w6058, w6067, w6068) -> (w6062:sgl)
                                n2905 = case shown="True" w6059 {
                                tunnel: w6062 -> [_ w6073]
                                tunnel: [0.0 w6073] -> w6057
                                frame False {
                                }
                                frame True {
                                }
                                }
                                n2906 = flat-sequence {
                                tunnel: w6056 -> [w6069]
                                tunnel: w6057 -> [w6071]
                                tunnel: w6056 -> [w6070]
                                frame #0 {
                                n2907 = call "prepAI_sealtest.vi"("samples per channel"=w6069) -> ()  [unwired: 2 in]
                                }
                                frame #1 {
                                n2908 = call "prepAO_sealtest.vi"("Vhold"=w6071, "samples per channel"=w6070) -> ()  [unwired: 1 in]
                                }
                                }
                                }
                              }
                            }
                            frame #5 {
                              n2909 = case shown="True" w6074 {
                                frame False {
                                }
                                frame True {
                                n2910 = stacked-sequence {
                                frame #0 {
                                n2911 = call "tempconfigAO.vi"("command"="get") -> ("Temp Config out"=w6081:T27)  [unwired: 1 in]
                                n2912 = Unbundle By Name(w6081) -> ("AO"=w6080:refnum<k21>[], "E_AO"=w6079:errorcluster[])
                                n2913 = for {
                                tunnel: w6080 -> [w6088] mode=indexing
                                tunnel: w6079 -> [w6087] mode=indexing
                                tunnel: [w6086] -> w6077 mode=indexing
                                tunnel: [w6085] -> w6076 mode=indexing
                                n2914 = call <vilib>:"DAQmx Start Task.vi"("task/channels in"=w6088, "error in"=w6087) -> ("task out"=w6086:refnum<k21>, "error out"=w6085:errorcluster)  [unwired: 12 in]
                                }
                                n2915 = call "tempconfigAO.vi"("command"="get") -> ("Temp Config out"=w6078:T27)  [unwired: 1 in]
                                n2916 = Bundle By Name(cluster=w6078, "AO"=w6077, "E_AO"=w6076) -> (w6075:T27)
                                n2917 = call "tempconfigAO.vi"("Temp Config in"=w6075, "command"="set") -> ()  [unwired: 1 out]
                                }
                                frame #1 {
                                n2918 = call "tempconfigAI.vi"("command"="get") -> ("Temp Config out"=w6090:T28)  [unwired: 1 in]
                                n2919 = Unbundle By Name(w6090) -> ("AI"=w6095:refnum<k21>, "E_AI"=w6096:errorcluster)
                                n2920 = call <vilib>:"DAQmx Start Task.vi"("task/channels in"=w6095, "error in"=w6096) -> ("task out"=w6097:refnum<k21>, "error out"=w6098:errorcluster)  [unwired: 12 in]
                                n2921 = call "tempconfigAI.vi"("command"="get") -> ("Temp Config out"=w6092:T28)  [unwired: 1 in]
                                n2922 = Bundle By Name(cluster=w6092, "AI"=w6097, "E_AI"=w6098) -> (w6094:T28)
                                n2923 = call "tempconfigAI.vi"("Temp Config in"=w6094, "command"="set") -> ()  [unwired: 1 out]
                                }
                                }
                                }
                              }
                            }
                          }
                        }
                        frame True {
                        }
                      }
                      n2924 = local read "readpatch"() -> (w5972:bool)
                      n2925 = Not(x=w5972) -> (.not. x?=w5971:bool)
                    }
                  }
                  frame #4 {
                    n2926 = call "tempconfigAO.vi"("command"="get") -> ("Temp Config out"=w6124:T27)  [unwired: 1 in]
                    n2927 = Unbundle By Name(w6124) -> ("AO"=w6123:refnum<k21>[], "E_AO"=w6122:errorcluster[])
                    n2928 = call "configuration.vi"("command"="get") -> ("config out"=w6105:T12)  [unwired: 2 in, 1 out]
                    n2929 = call "tempconfigAI.vi"("command"="get") -> ("Temp Config out"=w6111:T28)  [unwired: 1 in]
                    n2930 = Unbundle By Name(w6105) -> ("Device 1 sampleclock out"=w6102:tag, "Device 1 Starttrigger out"=w6101:tag)
                    n2931 = Unbundle By Name(w6111) -> ("AI"=w6112:refnum<k21>, "E_AI"=w6113:errorcluster)
                    n2932 = for {
                      tunnel: w6123 -> [w6128] mode=indexing
                      tunnel: w6122 -> [w6127] mode=indexing
                      tunnel: [w6126] -> w6118 mode=indexing
                      n2933 = call <vilib>:"DAQmx Stop Task.vi"("task/channels in"=w6128, "error in"=w6127) -> ("task out"=w6129:refnum<k21>, "error out"=w6130:errorcluster)  [unwired: 12 in]
                      n2934 = call <vilib>:"DAQmx Clear Task.vi"("task in"=w6129, "error in"=w6130) -> ("error out"=w6126:errorcluster)  [unwired: 13 in]
                    }
                    n2935 = call <vilib>:"DAQmx Stop Task.vi"("task/channels in"=w6112, "error in"=w6113) -> ("task out"=w6109:refnum<k21>, "error out"=w6108:errorcluster)  [unwired: 12 in]
                    n2936 = call <vilib>:"DAQmx Disconnect Terminals.vi"("source terminal"=tag "/Dev1/ai/SampleClock", "destination terminal"=w6102) -> ("error out"=w6099:errorcluster)  [unwired: 13 in]
                    n2937 = call <vilib>:"DAQmx Clear Task.vi"("task in"=w6109, "error in"=w6108) -> ("error out"=w6107:errorcluster)  [unwired: 13 in]
                    n2938 = call "tempconfigAO.vi"("command"="get") -> ("Temp Config out"=w6119:T27)  [unwired: 1 in]
                    n2939 = Bundle By Name(cluster=w6119, "E_AO"=w6118) -> (w6117:T27)
                    n2940 = call "tempconfigAI.vi"("command"="get") -> ("Temp Config out"=w6115:T28)  [unwired: 1 in]
                    n2941 = Bundle By Name(cluster=w6115, "E_AI"=w6107) -> (w6106:T28)
                    n2942 = call "tempconfigAO.vi"("Temp Config in"=w6117, "command"="set") -> ()  [unwired: 1 out]
                    n2943 = call <vilib>:"DAQmx Disconnect Terminals.vi"("source terminal"=tag "/Dev1/ai/StartTrigger", "destination terminal"=w6101, "error in"=w6099) -> ()  [unwired: 12 in, 1 out]
                    n2944 = call "tempconfigAI.vi"("Temp Config in"=w6106, "command"="set") -> ()  [unwired: 1 out]
                  }
                  frame #5 {
                    w6133 = T22 4 items=["no dialog", "OK message", "continue or stop message", "OK message + warnings", "continue/stop + warnings"] ("type of dialog (OK msg:1)")
                    n2945 = call "displayerrors.vi"() -> ("error IO"=w6132:errorcluster)
                    n2946 = call "zeropatch.vi"() -> ()  [unwired: 12 in]
                    n2947 = call <vilib>:"Simple Error Handler.vi"("type of dialog (OK msg:1)"=w6133, "error in (no error)"=w6132) -> ("error out"=w6131:errorcluster)  [unwired: 3 in, 4 out]
                    n2948 = call <vilib>:"Clear Errors.vi"("error in (no error)"=w6131) -> ()  [unwired: 5 in, 2 out]
                  }
                }
              }
            }
          }
          event "Current Clamp": Value Change {
            n2949 = event-data() -> ()  [unwired: 1 in, 6 out]
            n2950 = local read "Current Clamp"() -> (w6138:bool)
            n2951 = property on="Vholding (mV)" class="DigNum (strict)"("Caption.Text"="Ihold (pA)") -> ()  [unwired: 2 in, 2 out]
            n2952 = Not(x=w6138) -> (.not. x?=w6137:bool)
            n2953 = property on="Voltage Clamp" class="Bool (strict)"("Value"=w6137) -> ()  [unwired: 2 in, 2 out]
            n2954 = One Button Dialog(message="Have you switched the HEKA to CC and changed the external input cable?", button name ("OK")="Ok") -> ()  [unwired: 1 out]
          }
          event "Voltage Clamp": Value Change {
            n2955 = event-data() -> ()  [unwired: 1 in, 6 out]
            n2956 = local read "Voltage Clamp"() -> (w6143:bool)
            n2957 = Not(x=w6143) -> (.not. x?=w6142:bool)
            n2958 = property on="Current Clamp" class="Bool (strict)"("Value"=w6142) -> ()  [unwired: 2 in, 2 out]
            n2959 = One Button Dialog(message="Have you switched the HEKA to VC and changed the external input cable?", button name ("OK")="Ok") -> ()  [unwired: 1 out]
            n2960 = property on="Vholding (mV)" class="DigNum (strict)"("Caption.Text"="Vhold (mV)") -> ()  [unwired: 2 in, 2 out]
          }
          event "OCgain": Value Change {
            n2961 = event-data() -> ()  [unwired: 1 in, 6 out]
            n2962 = local read "OCgain"() -> (w6146:sgl)
            n2963 = Less?(x=w6146, y=0.3) -> (x < y?=w6144:bool)
            n2964 = case shown="True" w6144 {
              frame False {
                w6147 = 10.0 items=["0.1"=10.0, "10"=0.1] ("CC_ICgain")
                n2965 = local write "CC_ICgain"(w6147) -> ()
              }
              frame True {
                w6148 = 0.1 items=["0.1"=10.0, "10"=0.1] ("CC_ICgain")
                n2966 = local write "CC_ICgain"(w6148) -> ()
              }
            }
          }
          event "holdon": Value Change {
            n2967 = event-data() -> ()  [unwired: 1 in, 6 out]
            n2968 = stacked-sequence {
              frame #0 {
                n2969 = local read "Vholding (mV)"() -> (w6152:sgl)
                n2970 = local read "holdon"() -> (w6149:bool)
                n2971 = call "patchparameters.vi"("command"="get") -> ("Params out"=w6153:T14)  [unwired: 1 in]
                n2972 = Bundle By Name(cluster=w6153, "Vhold (mV)"=w6152, "holdon"=w6149) -> (w6150:T14)
                n2973 = call "patchparameters.vi"("Params in"=w6150, "command"="set") -> ()  [unwired: 1 out]
              }
              frame #1 {
                n2974 = call "zeropatch.vi"() -> ()  [unwired: 12 in]
              }
            }
          }
          event "Vholding (mV)": Value Change {
            n2975 = event-data() -> ()  [unwired: 1 in, 6 out]
            n2976 = local read "holdon"() -> (w6155:bool)
            n2977 = case shown="True" w6155 {
              frame False {
              }
              frame True {
                n2978 = stacked-sequence {
                  frame #0 {
                    n2979 = local read "Vholding (mV)"() -> (w6158:sgl)
                    n2980 = local read "holdon"() -> (w6159:bool)
                    n2981 = call "patchparameters.vi"("command"="get") -> ("Params out"=w6160:T14)  [unwired: 1 in]
                    n2982 = Bundle By Name(cluster=w6160, "Vhold (mV)"=w6158, "holdon"=w6159) -> (w6156:T14)
                    n2983 = call "patchparameters.vi"("Params in"=w6156, "command"="set") -> ()  [unwired: 1 out]
                  }
                  frame #1 {
                    n2984 = call "zeropatch.vi"() -> ()  [unwired: 12 in]
                  }
                }
              }
            }
          }
          event "AI channels": Value Change {
            n2985 = event-data() -> ()  [unwired: 1 in, 6 out]
            n2986 = local read "CI channels"() -> (w6169:i32[])
            n2987 = local read "AI channels"() -> (w6170:i32[])
            n2988 = call "configuration.vi"("command"="get") -> ("config out"=w6163:T12)  [unwired: 2 in, 1 out]
            n2989 = Unbundle By Name(w6163) -> ("CI names"=w6164:string[], "AI names"=w6165:string[])
            n2990 = for {
              tunnel: w6169 -> [w6175] mode=indexing
              tunnel: w6164 -> [w6176]
              tunnel: [w6174] -> w6166 mode=indexing
              n2991 = Index Array(array=w6176, index=w6175) -> (element=w6174:string)
            }
            n2992 = for {
              tunnel: w6170 -> [w6172] mode=indexing
              tunnel: w6165 -> [w6173]
              tunnel: [w6171] -> w6167 mode=indexing
              n2993 = Index Array(array=w6173, index=w6172) -> (element=w6171:string)
            }
            n2994 = Build Array (concatenate)(w6166, w6167) -> (w6168:string[])
            n2995 = property on="image1list" class="Ring (strict)"("Strings []"=w6168) -> ()  [unwired: 2 in, 2 out]
            n2996 = property on="image2list" class="Ring (strict)"("Strings []"=w6168) -> ()  [unwired: 2 in, 2 out]
          }
          event "CI channels": Value Change {
            n2997 = event-data() -> ()  [unwired: 1 in, 6 out]
            n2998 = local read "CI channels"() -> (w6184:i32[])
            n2999 = local read "AI channels"() -> (w6185:i32[])
            n3000 = call "configuration.vi"("command"="get") -> ("config out"=w6178:T12)  [unwired: 2 in, 1 out]
            n3001 = Unbundle By Name(w6178) -> ("CI names"=w6179:string[], "AI names"=w6180:string[])
            n3002 = for {
              tunnel: w6184 -> [w6190] mode=indexing
              tunnel: w6179 -> [w6191]
              tunnel: [w6189] -> w6181 mode=indexing
              n3003 = Index Array(array=w6191, index=w6190) -> (element=w6189:string)
            }
            n3004 = for {
              tunnel: w6185 -> [w6187] mode=indexing
              tunnel: w6180 -> [w6188]
              tunnel: [w6186] -> w6182 mode=indexing
              n3005 = Index Array(array=w6188, index=w6187) -> (element=w6186:string)
            }
            n3006 = Build Array (concatenate)(w6181, w6182) -> (w6183:string[])
            n3007 = property on="image1list" class="Ring (strict)"("Strings []"=w6183) -> ()  [unwired: 2 in, 2 out]
            n3008 = property on="image2list" class="Ring (strict)"("Strings []"=w6183) -> ()  [unwired: 2 in, 2 out]
          }
          event "setdatdir": Value Change {
            n3009 = event-data() -> ()  [unwired: 1 in, 5 out]
            n3010 = case shown="True" "setdatdir" {
              frame False {
              }
              frame True {
                n3011 = stacked-sequence {
                  frame #0 {
                    n3012 = local read "data dir"() -> (w6193:path)
                    n3013 = call "File Dialog"("start path"=w6193, "prompt"="Please select data directory...") -> ("selected path"=w6195:path, "cancelled"=w6194:bool, "error out"=w6196:errorcluster)  [unwired: 10 in, 1 out]
                    n3014 = case shown="False" w6194 {
                      tunnel: w6195 -> [w6204 _]
                      tunnel: w6196 -> [w6201 w6207]
                      tunnel: [w6199 w6207] -> w6198
                      frame False {
                        n3015 = local write "data dir"(w6204) -> ()
                        n3016 = call "configuration.vi"("error in"=w6201, "command"="get") -> ("Error out"=w6200:errorcluster, "config out"=w6206:T12)  [unwired: 1 in]
                        n3017 = Bundle By Name(cluster=w6206, "master data dir"=w6204) -> (w6205:T12)
                        n3018 = call "configuration.vi"("error in"=w6200, "config in"=w6205, "command"="set") -> ("Error out"=w6199:errorcluster)  [unwired: 1 out]
                      }
                      frame True {
                      }
                    }
                    n3019 = local write "status"(w6198) -> ()
                  }
                  frame #1 {
                    n3020 = property on="setdatdir" class="Bool (strict)"("Value"=FALSE ("setdatdir")) -> ()  [unwired: 2 in, 2 out]
                  }
                }
              }
            }
          }
          event "Shutter": Value Change {
            n3021 = event-data() -> ()  [unwired: 1 in, 5 out]
            n3022 = case shown="False" "Shutter" {
              frame False {
                n3023 = call "shuttercontrol.vi"("command"="close") -> ()  [unwired: 1 in, 1 out]
              }
              frame True {
                n3024 = call "shuttercontrol.vi"("command"="open") -> ()  [unwired: 1 in, 1 out]
              }
            }
          }
          event "ROI": Value Change {
            n3025 = event-data() -> ()  [unwired: 1 in, 5 out]
            n3026 = local read "ROI"() -> (w6212:bool)
            n3027 = case shown="True" w6212 {
              frame False {
              }
              frame True {
                n3028 = stacked-sequence {
                  frame #0 {
                    n3029 = local read "Square pixels"() -> (w6229:bool)
                    n3030 = local read "square matrix"() -> (w6228:bool)
                    n3031 = local read "Vx-max ref"() -> (w6234:dbl)
                    n3032 = local read "Vx-min ref"() -> (w6233:dbl)
                    n3033 = local read "Vy-min ref"() -> (w6230:dbl)
                    n3034 = local read "ypixels ref"() -> (w6232:i32)
                    n3035 = local read "Vy-max ref"() -> (w6231:dbl)
                    n3036 = local read "xpixels ref"() -> (w6235:i32)
                    n3037 = local read "Angle ref"() -> (w6227:dbl)
                    n3038 = local read "Colormap"() -> (w6236:i32)
                    n3039 = call "2pparameters.vi"("command"="get") -> ("params out"=w6239:T11)  [unwired: 1 in]
                    n3040 = Bundle By Name(cluster=w6239, "Xpixels Img"=w6235, "Vx-min Img"=w6233, "VX-max Img"=w6234, "Ypixels Img"=w6232, "Vy-min Img"=w6230, "Vy-max Img"=w6231, "Colormap"=w6236, "square pixels"=w6229, "square matrix"=w6228, "Angle Img"=w6227) -> (w6238:T11)
                    n3041 = call "2pparameters.vi"("Params in"=w6238, "command"="set") -> ()  [unwired: 1 out]
                    n3042 = local read "Vx-max draw"() -> (w6219:dbl)
                    n3043 = local read "Angle drawing"() -> (w6226:dbl)
                    n3044 = local read "Vx-min draw"() -> (w6220:dbl)
                    n3045 = local read "Vy-min draw"() -> (w6223:dbl)
                    n3046 = local read "ypixels draw"() -> (w6221:dbl)
                    n3047 = local read "Vy-max draw"() -> (w6222:dbl)
                    n3048 = local read "Square pixels"() -> (w6224:bool)
                    n3049 = local read "square matrix"() -> (w6225:bool)
                    n3050 = local read "xpixels draw"() -> (w6218:dbl)
                    n3051 = local read "Colormap"() -> (w6217:i32)
                    n3052 = call "2pparameters.vi"("command"="get") -> ("params out"=w6214:T11)  [unwired: 1 in]
                    n3053 = Bundle By Name(cluster=w6214, "Xpixels"=w6218, "Vxminref"=w6220, "Vxmaxref"=w6219, "Ypixels"=w6221, "Vyminref"=w6223, "Vymaxref"=w6222, "Colormap"=w6217, "square pixels"=w6224, "square matrix"=w6225, "Angle draw"=w6226) -> (w6215:T11)
                    n3054 = call "2pparameters.vi"("Params in"=w6215, "command"="set") -> ()  [unwired: 1 out]
                  }
                  frame #1 {
                    n3055 = Current VI's Path() -> (path=w6250:path)
                    n3056 = Strip Path(path=w6250) -> (stripped path=w6251:path)  [unwired: 1 out]
                    n3057 = Build Path(base path=w6251, name or relative path="subVIs\\Image\\SetROI_v3.vi") -> (appended path=w6249:path)
                    n3058 = call <vilib>:"Set Busy.vi"() -> ("error out"=w6247:errorcluster)  [unwired: 10 in, 1 out]
